vi "Resolve VI Path.vi"(8 "error in (no error)":errorcluster, 10 "Library Paths (.lvlibp, .lvlib)":path[](array[path]), 11 "Qualified Name (lvlibp|lvlib[:vi])":string) -> (0 "error out":errorcluster, 2 "Exists?":bool, 3 "VI Path":path)   [LabVIEW 2022 SP3, in "Shared.lvlib"]
uses:
  Shared.lvlib
  <vilib>/Utility/LVLibp/NI_PackedLibraryUtility.lvlib
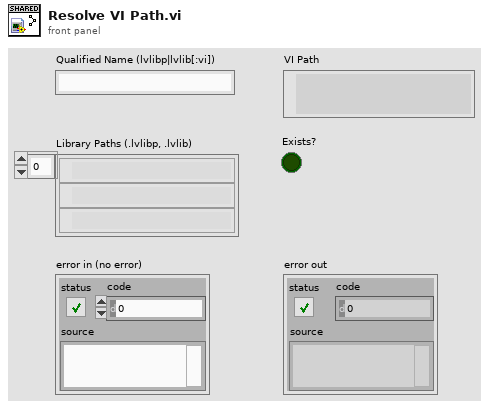
[diagram p1: front panel]
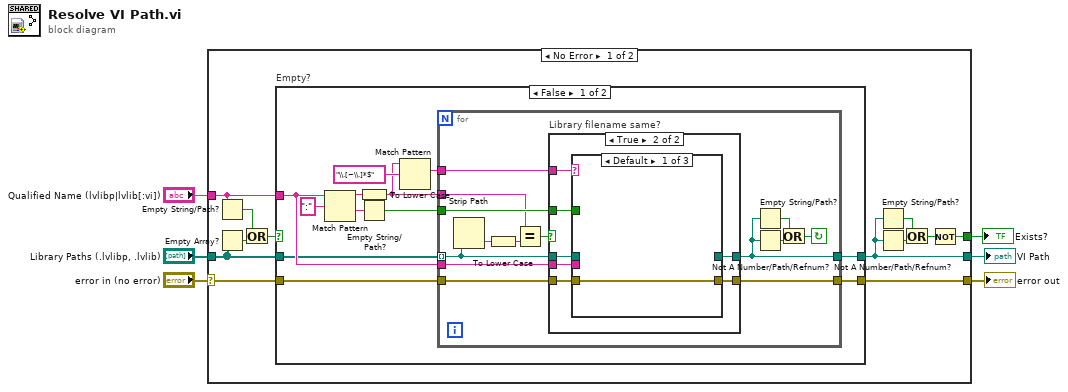
[diagram p0: block diagram]
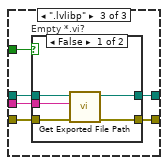
[diagram p4: hidden frame]
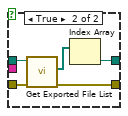
[diagram p5: hidden frame]
diagram:
  n1 = case shown="No Error" "error in (no error)" {
    selector: "error in (no error)" -> [w18 w72]
    tunnel: "Qualified Name (lvlibp|lvlib[:vi])" -> [w16 _]
    tunnel: [w17 w72] -> w4
    tunnel: "Library Paths (.lvlibp, .lvlib)" -> [w15 _]
    tunnel: [w9 _] -> w2
    tunnel: [w7 _] -> w1
    frame No Error {
      n2 = Empty String/Path?(string/path=w16) -> (empty?=w14:bool)
      n3 = Empty Array?(array=w15) -> (empty?=w13:bool)
      n4 = Or(x=w14, y=w13) -> (x .or. y?=w12:bool)
      n5 = case "Empty?" shown="False" w12 {
        tunnel: [w25 _] -> w9
        tunnel: w16 -> [w24 _]
        tunnel: w15 -> [w23 _]
        tunnel: w18 -> [w20 w71]
        tunnel: [w19 w71] -> w17
        frame False {
          n6 = Match Pattern(string=w24, regular expression=":") -> (before substring=w28:string, after substring=w27:string)  [unwired: 1 in, 2 out]
          n7 = To Lower Case(string=w28) -> (all lower case string=w22:string)
          n8 = Empty String/Path?(string/path=w27) -> (empty?=w26:bool)
          n9 = Match Pattern(string=w22, regular expression="\\.[~\\.]*$") -> (match substring=w21:string)  [unwired: 4 out]
          n10 = for {
            tunnel: w24 -> [w44]
            tunnel: w26 -> [w43]
            tunnel: [w35] -> w25
            tunnel: w21 -> [w39]
            tunnel: w23 -> [w42] mode=indexing
            tunnel: w22 -> [w33]
            tunnel: w20 -> [w32]
            tunnel: [w31] -> w19
            stop <- w34 continue-if-true
            n11 = Strip Path(path=w42) -> (name=w41:string)  [unwired: 1 out]
            n12 = To Lower Case(string=w41) -> (all lower case string=w40:string)
            n13 = Equal?(x=w33, y=w40) -> (x = y?=w38:bool)
            n14 = case "Library filename same?" shown="True" w38 {
              tunnel: w44 -> [_ w51]
              tunnel: w43 -> [_ w49]
              tunnel: [_ w50] -> w35
              tunnel: w42 -> [_ w52]
              tunnel: w39 -> [_ w48]
              tunnel: w32 -> [w45 w47]
              tunnel: [w45 w46] -> w31
              frame False {
              }
              frame True {
                n15 = case shown="Default" w48 {
                  tunnel: w52 -> [_ _ w60]
                  tunnel: w51 -> [_ _ w59]
                  tunnel: [_ _ w58] -> w50
                  tunnel: w49 -> [_ _ w57]
                  tunnel: w47 -> [w53 w54 w56]
                  tunnel: [w53 w54 w55] -> w46
                  frame Default {
                  }
                  frame ".lvlib" {
                    # "#ToDo"
                  }
                  frame ".lvlibp" {
                    n16 = case "Empty *.vi?" shown="False" w57 {
                      tunnel: w60 -> [w65 w70]
                      tunnel: w59 -> [w64 _]
                      tunnel: [w63 w68] -> w58
                      tunnel: [w62 w67] -> w55
                      tunnel: w56 -> [w61 w66]
                      frame False {
                        n17 = call <vilib>:"Get Exported File Path.vi"("error in (no error)"=w61, "qualified name"=w64, "packed library path"=w65) -> ("error out"=w62:errorcluster, "path"=w63:path)  [unwired: 7 in]
                      }
                      frame True {
                        n18 = call <vilib>:"Get Exported File List.vi"("error in (no error)"=w66, "packed library path"=w70) -> ("error out"=w67:errorcluster, "paths"=w69:path[])  [unwired: 7 in, 1 out]
                        n19 = Index Array(array=w69) -> (element=w68:path)  [unwired: 1 in]
                      }
                    }
                  }
                }
              }
            }
            n20 = Empty String/Path?(string/path=w35) -> (empty?=w36:bool)
            n21 = Not A Number/Path/Refnum?(number/path/refnum=w35) -> (NaN/Path/Refnum?=w37:bool)
            n22 = Or(x=w36, y=w37) -> (x .or. y?=w34:bool)
          }
        }
        frame True {
        }
      }
      n23 = Empty String/Path?(string/path=w9) -> (empty?=w11:bool)
      n24 = Not A Number/Path/Refnum?(number/path/refnum=w9) -> (NaN/Path/Refnum?=w10:bool)
      n25 = Or(x=w11, y=w10) -> (x .or. y?=w8:bool)
      n26 = Not(x=w8) -> (.not. x?=w7:bool)
    }
    frame Error {
    }
  }
  "error out" <- w4
  "VI Path" <- w2
  "Exists?" <- w1
